vi "Keyence.Main.Tune.Init.vi"(8 "error in":errorcluster, 10 "Bank":u8, 11 "Data in":T1={"Status"={"State"=enum."Init", "Ref"=refnum, "Bank"=0, "Version"="", "Model"="", "EndTS"=timestamp(0 s since 1904-01-01), "ImgPath"=path "", "Tuned"=FALSE}, "Sets"={"IP"="192.168.2.1", "Timeout_ms"=5000, "Retries"=0, "ReconnectPeriod_s"=0, "ResetPeriod_s"=0, "ReadImg"=FALSE}, "Code"={"text"="", "status"=FALSE, "corners"=[], "level"=0, "class"="", "path"=path ""}}) -> (0 "error out":errorcluster, 2 "started":bool, 3 "Data out":T1={"Status"={"State"=enum."Init", "Ref"=refnum, "Bank"=0, "Version"="", "Model"="", "EndTS"=timestamp(0 s since 1904-01-01), "ImgPath"=path "", "Tuned"=FALSE}, "Sets"={"IP"="192.168.2.1", "Timeout_ms"=5000, "Retries"=0, "ReconnectPeriod_s"=0, "ResetPeriod_s"=0, "ReadImg"=FALSE}, "Code"={"text"="", "status"=FALSE, "corners"=[], "level"=0, "class"="", "path"=path ""}})   [LabVIEW 2015]
uses:
  Keyence.Data.ctl
  Keyence.Data.Status.ctl
  Keyence.Data.Status.State.ctl
  Keyence.Data.Sets.ctl
  LowLevel/Keyence.CodeDetails.ctl
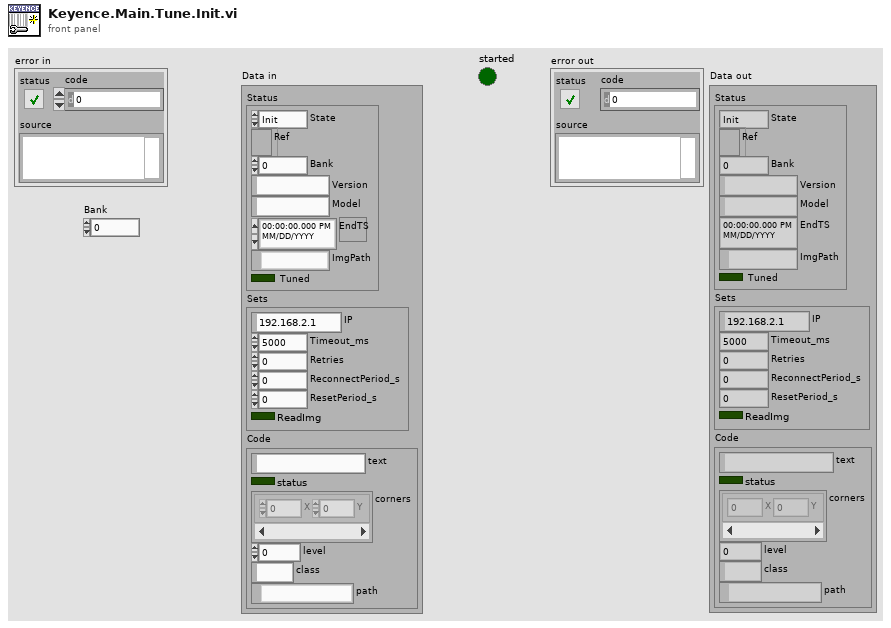
[diagram p1: front panel]
types:
  T1 = typedef "Keyence.Data.ctl" = cluster{"Status":T2, "Sets":T4, "Code":T5}
  T2 = typedef "Keyence.Data.Status.ctl" = cluster{"State":T3, "Ref":refnum<k5>, "Bank":u8, "Version":string, "Model":string, "EndTS":timestamp, "ImgPath":path, "Tuned":bool}
  T3 = typedef "Keyence.Data.Status.State.ctl" = enum16{"First", "Init", "Reset", "Idle", "Scan", "Tune"}
  T4 = typedef "Keyence.Data.Sets.ctl" = cluster{"IP":string, "Timeout_ms":i32, "Retries":i32, "ReconnectPeriod_s":i32, "ResetPeriod_s":i32, "ReadImg":bool}
  T5 = typedef "Keyence.CodeDetails.ctl" = cluster{"text":string, "status":bool, "corners":cluster{"X":i32, "Y":i32}[], "level":u8, "class":string, "path":path}
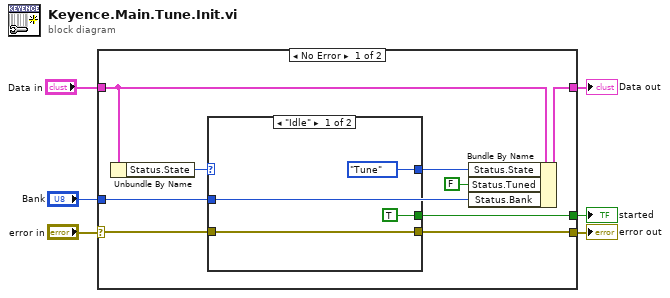
[diagram p0: block diagram]
diagram:
  n1 = case shown="No Error" "error in" {
    selector: "error in" -> [w11 w22]
    tunnel: [w13 w22] -> w3
    tunnel: "Data in" -> [w14 w21]
    tunnel: [w15 w21] -> w4
    tunnel: "Bank" -> [w7 _]
    tunnel: [w9 _] -> w1
    frame No Error {
      n2 = Unbundle By Name(w14) -> ("Status.State"=w12:T3)
      n3 = case shown="\"Idle\"" w12 {
        selector: w12 -> [_ w20]
        tunnel: w11 -> [w17 w19]
        tunnel: [w17 w19] -> w13
        tunnel: [Keyence.Data.Status.State."Tune" ("Status.State") w20] -> w10
        tunnel: [TRUE _] -> w9
        tunnel: w7 -> [_ _]
        frame "Idle" {
        }
        frame Default {
        }
      }
      n4 = Bundle By Name(cluster=w14, "Status.State"=w10, "Status.Tuned"=FALSE, "Status.Bank"=w7) -> (w15:T1)
    }
    frame Error {
    }
  }
  "error out" <- w3
  "Data out" <- w4
  "started" <- w1
